vi "Calibrate.vi"(7 "Enable Store Calibration (F: Disable)":bool, 8 "error in (no error)":errorcluster, 9 "Calibration Message ()":string, 10 "Calibration Value (0)":dbl, 11 "VISA resource name":refnum<visa-resource-name>) -> (0 "error out":errorcluster, 2 "Calibration Result":bool, 3 "VISA resource name out":refnum<visa-resource-name>)   [LabVIEW 2020, in "Agilent 3446X Series.lvlib"]
doc: "Performs a calibration using the calibration value based on the function and range.\n\n<B>Note(s):</B>\n1. A short must be applied for the resistance and voltage measurement functions, and the inputs must be open for the current measurement functions.\n2. You must unsecure the instrument to calibrate it or to change the calibration string or security code."
uses:
  Agilent 3446X Series.lvlib
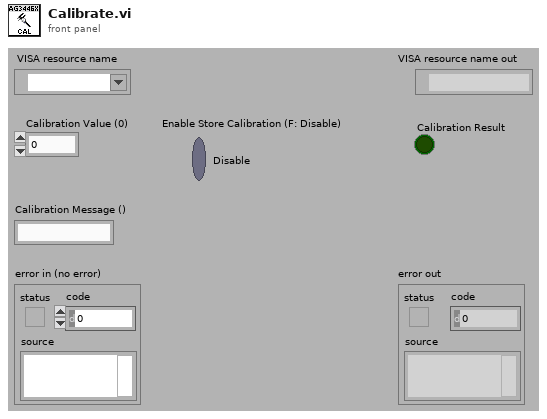
[diagram p1: front panel]
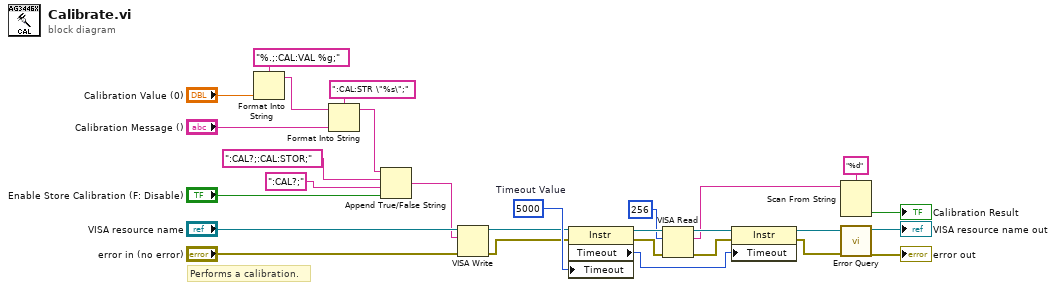
[diagram p0: block diagram]
diagram:
  w19 = u32 5000  # Timeout Value
  # "Performs a calibration."
  n1 = Format Into String(format string="%.;:CAL:VAL %g;", "Calibration Value (0)") -> (resulting string=w26:string)  [unwired: 2 in, 1 out]
  n2 = Format Into String(format string=":CAL:STR \"%s\";", initial string=w26, "Calibration Message ()") -> (resulting string=w4:string)  [unwired: 1 in, 1 out]
  n3 = Append True/False String(1:"Enable Store Calibration (F: Disable)", 2:":CAL?;" ("false string"), 3:":CAL?;:CAL:STOR;", 4:w4) -> (0:w2:string)
  n4 = VISA Write(VISA resource name="VISA resource name", write buffer=w2, error in (no error)="error in (no error)") -> (VISA resource name out=w10:refnum<visa-resource-name>, error out=w9:errorcluster)  [unwired: 1 out]
  n5 = property class="Instr"(reference=w10, error in=w9, "Timeout"=w19) -> (reference out=w18:refnum<visa-resource-name>, error out=w17:errorcluster, "Timeout"=w13:u32)
  n6 = VISA Read(VISA resource name=w18, byte count=u32 256, error in (no error)=w17) -> (VISA resource name out=w15:refnum<visa-resource-name>, read buffer=w11:string, error out=w14:errorcluster)  [unwired: 1 out]
  n7 = property class="Instr"(reference=w15, error in=w14, "Timeout"=w13) -> (reference out=w8:refnum<visa-resource-name>, error out=w7:errorcluster)
  n8 = Scan From String(format string="%d", input string=w11) -> (output 1=→"Calibration Result":bool)  [unwired: 2 in, 4 out]
  n9 = call "Error Query.vi"("error in (no error)"=w7, "VISA resource name"=w8) -> ("error out"=→"error out":errorcluster, "VISA resource name out"=→"VISA resource name out":refnum<visa-resource-name>)  [unwired: 8 out]
